vi "FT-IR EVID SysLog.vi"(10 "Anzahl":i32, 11 "Startadresse":i32) -> (2 "Anzahl out":i32, 3 "Startadresse out":i32)   [LabVIEW 2020, in "FT-IR.lvlib"]
uses:
  FT-IR.lvlib
  Aktionen EVID-Codes.ctl
  SysLog/SysLog Interface.ctl
  SysLog/SysLog.lvlib
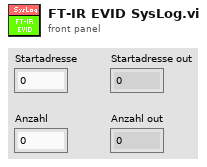
[diagram p1: front panel]
types:
  T1 = typedef "FT-IR.lvlib/Aktionen EVID-Codes.ctl" = enum16{"lesen", "setzen", "laden", "speichern", "1Hz/5Hz", "Smoothing", "Rolling Average"}
  T2 = typedef "SysLog.lvlib/SysLog Interface.ctl" = cluster{"FehlermeldungsCode":i32, "ErfolgsmeldungsCode":i32, "ParameterListenString":string, "Anzeige":bool, "SysLogIcon":enum16{"OK", "Warnung", "Fehler"}, "intern":bool}
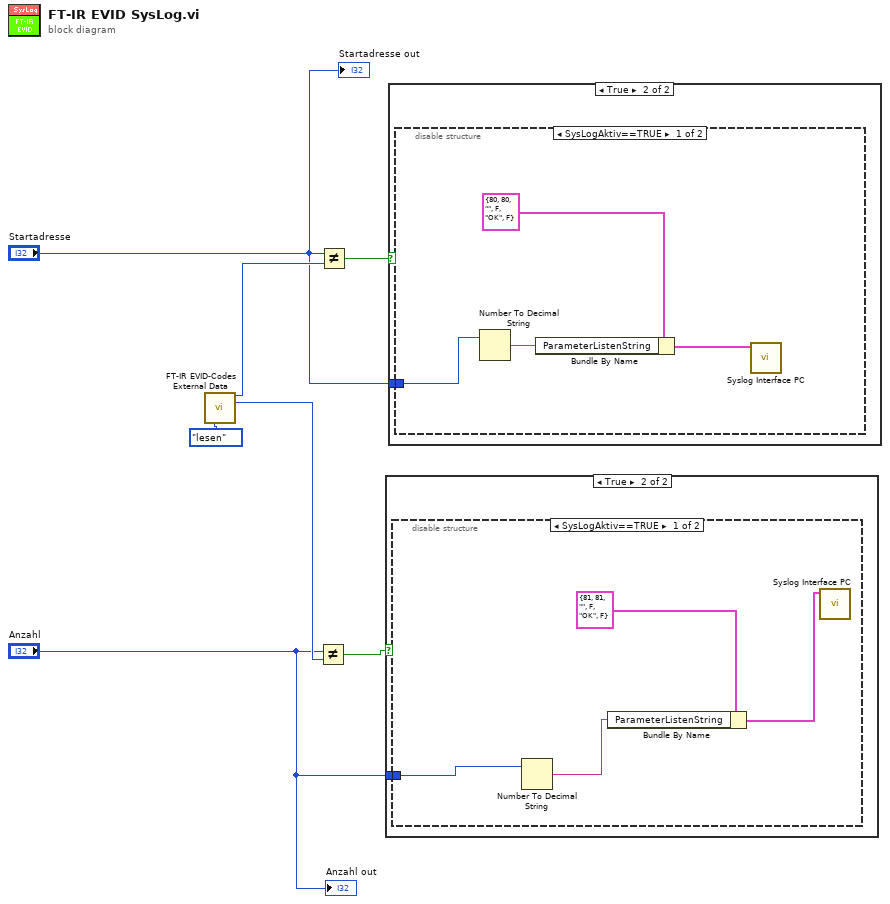
[diagram p0: block diagram]
diagram:
  n1 = call "FT-IR EVID-Codes External Data.vi"("Aktionen"=Aktionen_EVID-Codes."lesen") -> ("Startadresse"=w4:i32, "Anzahl"=w3:i32)  [unwired: 9 in, 4 out]
  n2 = Not Equal?(x="Anzahl", y=w3) -> (x != y?=w6:bool)
  n3 = Not Equal?(x="Startadresse", y=w4) -> (x != y?=w5:bool)
  n4 = case shown="True" w6 {
    tunnel: "Anzahl" -> [_ w8]
    frame False {
    }
    frame True {
      n5 = disable-structure shown="SysLogAktiv==TRUE" {
        disable-tunnel: w8 -> [w12 _]
        frame condition #0 (active) {
          n6 = Number To Decimal String(number=w12) -> (decimal integer string=w10:string)  [unwired: 1 in]
          n7 = Bundle By Name(cluster=T2 {"FehlermeldungsCode"=81, "ErfolgsmeldungsCode"=81, "ParameterListenString"="", "Anzeige"=FALSE, "SysLogIcon"=enum."OK", "intern"=FALSE} ("Cluster (in)"), "ParameterListenString"=w10) -> (w9:T2)
          n8 = call "Syslog Interface PC.vi"("Cluster (in)"=w9) -> ()  [unwired: 10 in, 1 out]
        }
        frame condition #1 {
        }
      }
    }
  }
  n9 = case shown="True" w5 {
    tunnel: "Startadresse" -> [_ w13]
    frame False {
    }
    frame True {
      n10 = disable-structure shown="SysLogAktiv==TRUE" {
        disable-tunnel: w13 -> [w17 _]
        frame condition #0 (active) {
          n11 = Number To Decimal String(number=w17) -> (decimal integer string=w15:string)  [unwired: 1 in]
          n12 = Bundle By Name(cluster=T2 {"FehlermeldungsCode"=80, "ErfolgsmeldungsCode"=80, "ParameterListenString"="", "Anzeige"=FALSE, "SysLogIcon"=enum."OK", "intern"=FALSE} ("Cluster (in)"), "ParameterListenString"=w15) -> (w14:T2)
          n13 = call "Syslog Interface PC.vi"("Cluster (in)"=w14) -> ()  [unwired: 10 in, 1 out]
        }
        frame condition #1 {
        }
      }
    }
  }
  "Startadresse out" <- "Startadresse"
  "Anzahl out" <- "Anzahl"
